vi "SSC DCPower Configure Output Resistance Array.vi"(0 "DCPower SSC in":T1[](array[typedef]), 5 "Output Resistance (Ohms)":dbl[](array[numeric]) format="%#_6p", 11 "error in":errorcluster) -> (4 "DCPower SSC out":T1[](array[typedef]), 15 "error out":errorcluster)   [LabVIEW 2020]
doc: "This VI configures output resistance on the channels."
uses:
  SSC DCPower.ctl
  575ce6e6-a650-4577-b389-4142566cffc2.vi
  <vilib>/Utility/error.llb/Error Cluster From Error Code.vi
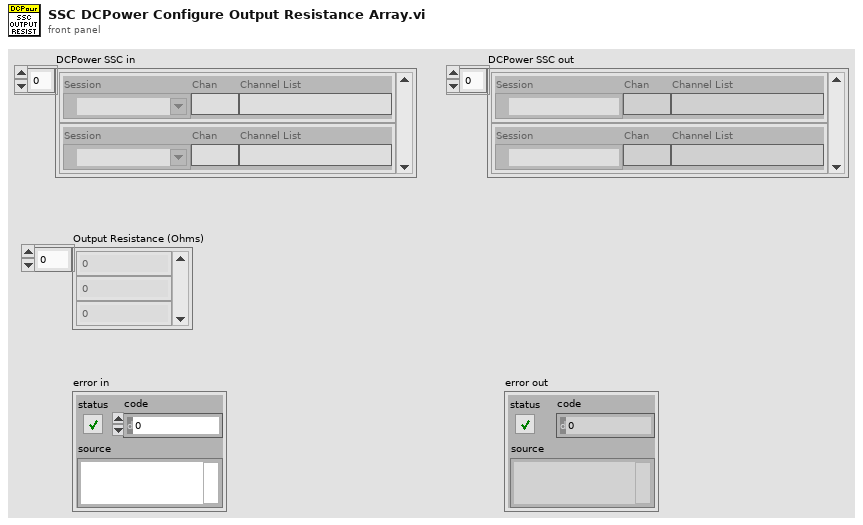
[diagram p1: front panel]
types:
  T1 = typedef "SSC DCPower.ctl" = cluster{"Session":refnum<k15>, "Chan":string, "Channel List":string}
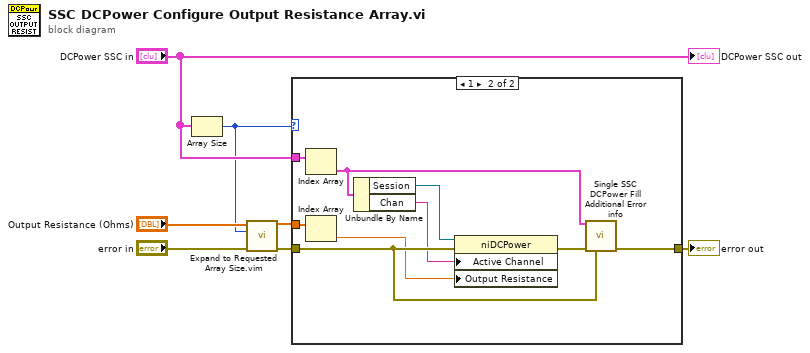
[diagram p0: block diagram]
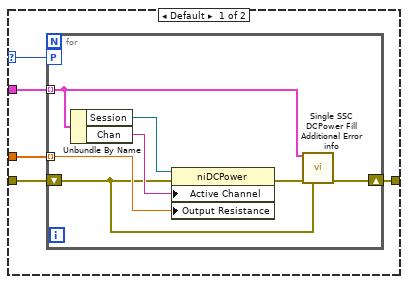
[diagram p2: hidden frame]
diagram:
  n1 = Array Size(array="DCPower SSC in") -> (size(s)=w1:i32)
  n2 = call "Expand to Requested Array Size.vim"("Data In"="Output Resistance (Ohms)", "Requested Size"=w1, "error in"="error in") -> ("Data Out"=w2:dbl[], "error out"=w4:errorcluster)  [unwired: 11 in]
  n3 = case shown="1" w1 {
    selector: w1 -> [w9 _]
    tunnel: [w12 w28] -> w7
    tunnel: w2 -> [w11 w27]
    tunnel: w4 -> [w10 w26]
    tunnel: "DCPower SSC in" -> [w8 w25]
    frame Default {
      n4 = for {
        tunnel: w8 -> [w14] mode=indexing
        tunnel: w11 -> [w18] mode=indexing
        workers-P: w9 -> [_]
        shift-right: [w15] -> w12
        shift-left: w10 -> [w13]
        n5 = Unbundle By Name(w14) -> ("Session"=w17:refnum<k15>, "Chan"=w16:string)
        n6 = property class="niDCPower"(reference=w17, error in=w13, "Active Channel"=w16, "Output Resistance"=w18) -> (error out=w19:errorcluster)  [unwired: 1 out]
        n7 = call "Single SSC DCPower Fill Additional Error info.vi"("DCPower SSC in"=w14, "error in"=w19, "previous error in"=w13) -> ("error out"=w15:errorcluster)  [unwired: 12 in]
      }
    }
    frame 1 {
      n8 = Index Array(array=w25) -> (element=w21:T1)  [unwired: 1 in]
      n9 = Index Array(array=w27) -> (element=w20:dbl)  [unwired: 1 in]
      n10 = Unbundle By Name(w21) -> ("Session"=w23:refnum<k15>, "Chan"=w22:string)
      n11 = property class="niDCPower"(reference=w23, error in=w26, "Active Channel"=w22, "Output Resistance"=w20) -> (error out=w24:errorcluster)  [unwired: 1 out]
      n12 = call "Single SSC DCPower Fill Additional Error info.vi"("DCPower SSC in"=w21, "error in"=w24, "previous error in"=w26) -> ("error out"=w28:errorcluster)  [unwired: 12 in]
    }
  }
  "error out" <- w7
  "DCPower SSC out" <- "DCPower SSC in"
